vi "Get Last Week Stats.vi"(11 "WPC Stats":T1[][](array[typedef]) {"Date Updated" format="%<%m/%d/%Y>T"}) -> (3 "Last Week's Stats":T1[](array[typedef]) {"Date Updated" format="%<%m/%d/%Y>T"})   [LabVIEW 2021]
uses:
  WPC Player and Financial Stats.ctl
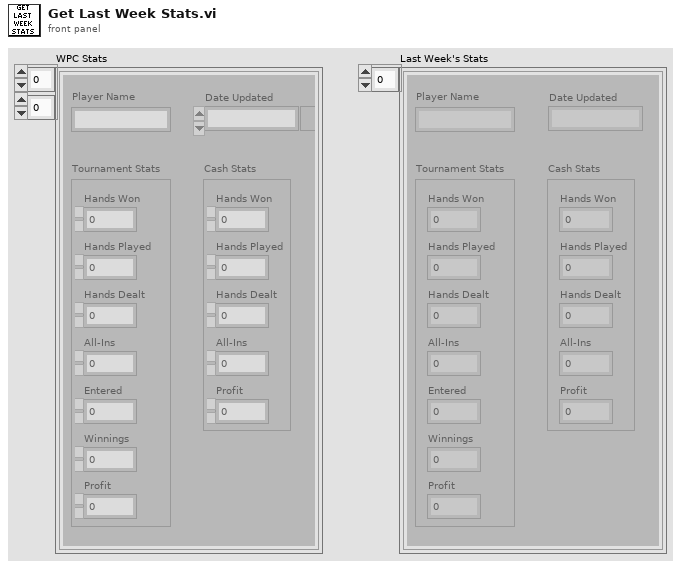
[diagram p1: front panel]
types:
  T1 = typedef "WPC Player and Financial Stats.ctl" = cluster{"Player Name":string, "Date Updated":timestamp, "Tournament Stats":cluster{"Hands Won":i32, "Hands Played":i32, "Hands Dealt":i32, "All-Ins":i32, "Entered":i32, "Winnings":dbl, "Profit":dbl}, "Cash Stats":cluster{"Hands Won":i32, "Hands Played":i32, "Hands Dealt":i32, "All-Ins":i32, "Profit":dbl}}
  T2 = cluster{"Hands Won":i32, "Hands Played":i32, "Hands Dealt":i32, "All-Ins":i32, "Entered":i32, "Winnings":dbl, "Profit":dbl}
  T3 = cluster{"Hands Won":i32, "Hands Played":i32, "Hands Dealt":i32, "All-Ins":i32, "Profit":dbl}
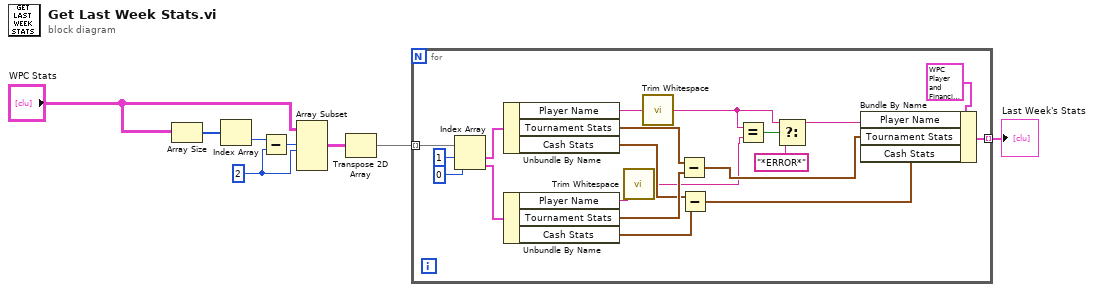
[diagram p0: block diagram]
diagram:
  w5 = 2 ("length")
  n1 = Array Size(array="WPC Stats") -> (size(s)=w2:i32[])
  n2 = Index Array(array=w2) -> (element=w6:i32)  [unwired: 1 in]
  n3 = Subtract(x=w6, y=w5) -> (x-y=w4:i32)
  n4 = Array Subset(array="WPC Stats", index (row)=w4, length (row)=w5) -> (w7:T1[][])  [unwired: 2 in]
  n5 = Transpose 2D Array(2D array=w7) -> (transposed array=w8:T1[][])
  n6 = for {
    tunnel: w8 -> [w28] mode=indexing
    tunnel: [w19] -> w1 mode=indexing
    n7 = Index Array(array=w28, index #1=1 ("index"), index #2=0 ("index")) -> (element #1=w25:T1, element #2=w18:T1)
    n8 = Unbundle By Name(w25) -> ("Player Name"=w22:string, "Tournament Stats"=w17:T2, "Cash Stats"=w15:T3)
    n9 = Unbundle By Name(w18) -> ("Player Name"=w24:string, "Tournament Stats"=w16:T2, "Cash Stats"=w14:T3)
    n10 = call <vilib>:"Trim Whitespace.vi"("string"=w24) -> ("trimmed string"=w9:string)  [unwired: 1 in]
    n11 = call <vilib>:"Trim Whitespace.vi"("string"=w22) -> ("trimmed string"=w10:string)  [unwired: 1 in]
    n12 = Subtract(x=w17, y=w16) -> (x-y=w13:T2)
    n13 = Subtract(x=w15, y=w14) -> (x-y=w12:T3)
    n14 = Equal?(x=w10, y=w9) -> (x = y?=w23:bool)
    n15 = Select(t=w10, s=w23, f="*ERROR*") -> (s? t:f=w20:string)
    n16 = Bundle By Name(cluster=T1 {"Player Name"="", "Date Updated"=timestamp(0 s since 1904-01-01), "Tournament Stats"={"Hands Won"=0, "Hands Played"=0, "Hands Dealt"=0, "All-Ins"=0, "Entered"=0, "Winnings"=0.0, "Profit"=0.0}, "Cash Stats"={"Hands Won"=0, "Hands Played"=0, "Hands Dealt"=0, "All-Ins"=0, "Profit"=0.0}} ("WPC Player Stats"), "Player Name"=w20, "Tournament Stats"=w13, "Cash Stats"=w12) -> (w19:T1)
  }
  "Last Week's Stats" <- w1
